vi "A1 Packet.vi"(9 "All Zeros?":bool, 10 "0x0D?":bool, 11 "DUT Serial #":i32) -> (3 "Array":u8[](array[numeric]))   [LabVIEW 2015]
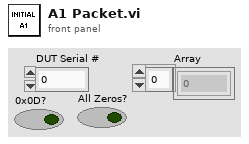
[diagram p1: front panel]
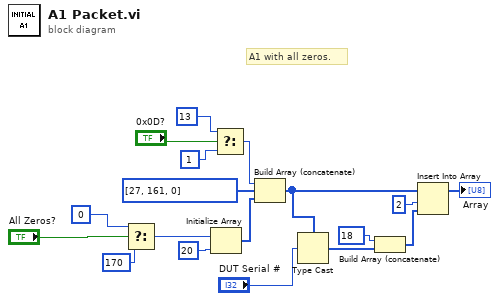
[diagram p0: block diagram]
diagram:
  # "A1 with all zeros."
  n1 = Select(t=u8 0, s="All Zeros?", f=u8 170) -> (s? t:f=w6:u8)
  n2 = Initialize Array(w6, 20 ("dimension size")) -> (w13:u8[])
  n3 = Select(t=u8 13, s="0x0D?", f=u8 1) -> (s? t:f=w2:u8)
  n4 = Build Array (concatenate)(w2, u8[] [27, 161, 0] ("initialized array"), w13) -> (w12:u8[])
  n5 = Type Cast(type=w12, x="DUT Serial #") -> (*(type *) &x=w14:u8[])
  n6 = Build Array (concatenate)(u8 18, w14) -> (w10:u8[])
  n7 = Insert Into Array(array=w12, index=2, new element=w10) -> (→"Array":u8[])
